vi "FindNode.vi"(5 "VI":string, 9 "VI_AST in":refnum<class "VI_Hierarchy.lvclass">) -> (3 "VI_AST out":refnum<class "VI_Hierarchy.lvclass">, 4 "index":i32)   [LabVIEW 2014, in "VI_Hierarchy.lvclass"]
uses:
  VI_Hierarchy.lvclass
  VI_Hierarchy.lvclass/VI_Hierarchy.ctl
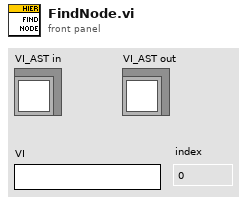
[diagram p1: front panel]
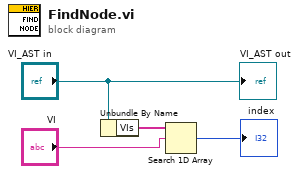
[diagram p0: block diagram]
diagram:
  n1 = Unbundle By Name("VI_AST in") -> ("VIs"=w3:string[])
  n2 = Search 1D Array(1D array=w3, element="VI") -> (index of element=→"index":i32)  [unwired: 1 in]
  "VI_AST out" <- "VI_AST in"
